vi "color_table_.vi"(9 "N":i32, 10 "Color 2":u32(colorbox), 11 "Color 1":u32(colorbox)) -> (3 "Color Table (element 0=color 1, element N-1=color 2)":u32[](array[colorbox]))   [LabVIEW 2020]
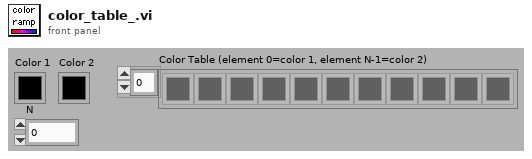
[diagram p1: front panel]
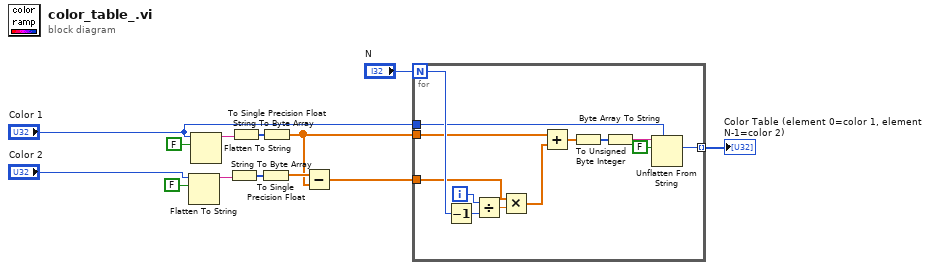
[diagram p0: block diagram]
diagram:
  n1 = Flatten To String(anything="Color 2", prepend array or string size? (T)=FALSE) -> (data string=w11:string)  [unwired: 2 in, 2 out]
  n2 = Flatten To String(anything="Color 1", prepend array or string size? (T)=FALSE) -> (data string=w12:string)  [unwired: 2 in, 2 out]
  n3 = String To Byte Array(string=w11) -> (unsigned byte array=w6:u8[])
  n4 = String To Byte Array(string=w12) -> (unsigned byte array=w7:u8[])
  n5 = To Single Precision Float(number=w6) -> (single precision float=w5:sgl[])
  n6 = To Single Precision Float(number=w7) -> (single precision float=w3:sgl[])
  n7 = Subtract(x=w5, y=w3) -> (x-y=w4:sgl[])
  n8 = for {
    N: "N" -> [w24]
    tunnel: w4 -> [w22]
    tunnel: w3 -> [w20]
    tunnel: "Color 1" -> [w15]
    tunnel: [w14] -> w1 mode=indexing
    i -> [w25]
    n9 = Decrement(x=w24) -> (x-1=w26:i32)
    n10 = Divide(x=w25, y=w26) -> (x/y=w23:dbl)
    n11 = Multiply(x=w22, y=w23) -> (x*y=w21:dbl[])
    n12 = Add(x=w20, y=w21) -> (x+y=w19:dbl[])
    n13 = To Unsigned Byte Integer(number=w19) -> (unsigned 8bit integer=w18:u8[])
    n14 = Byte Array To String(unsigned byte array=w18) -> (string=w17:string)
    n15 = Unflatten From String(type=w15, binary string=w17, data includes array or string size? (T)=FALSE) -> (value=w14:u32)  [unwired: 2 in, 2 out]
  }
  "Color Table (element 0=color 1, element N-1=color 2)" <- w1
